vi "Refactor Object for Library Rename.vi"(8 "error in (no error)":errorcluster, 10 "rename data":T2, 11 "object reference in":refnum<vi>) -> (0 "error out":errorcluster, 1 "refactored dependency":bool, 2 "refactor result":T1, 3 "object reference out":refnum<vi>)   [LabVIEW 2021, in "MeasurementService Editor.lvlib"]
uses:
  MeasurementService Editor.lvlib
  Refactor Object Result.ctl
  Rename Refactor Mapping Info.ctl
  Rename Refactor Data.ctl
  Rename String Mapping.ctl
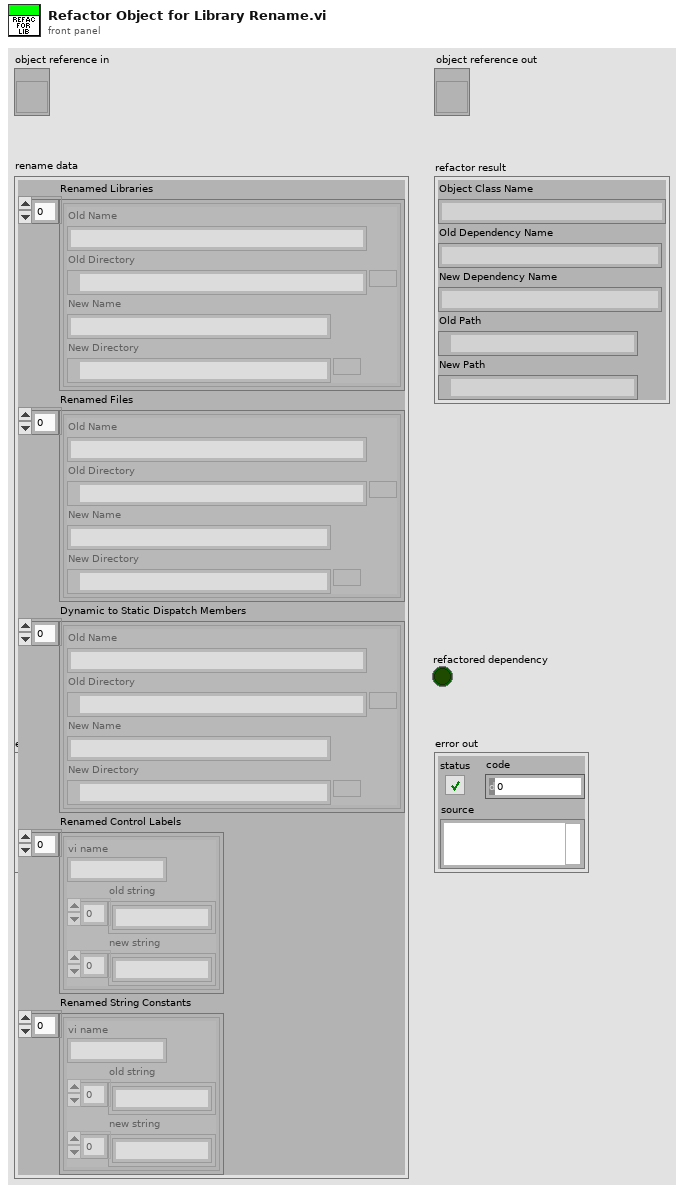
[diagram p1: front panel]
types:
  T1 = typedef "MeasurementService Editor.lvlib/Refactor Object Result.ctl" = cluster{"Object Class Name":string, "Old Dependency Name":string, "New Dependency Name":string, "Old Path":path, "New Path":path}
  T2 = typedef "MeasurementService Editor.lvlib/Rename Refactor Data.ctl" = cluster{"Renamed Libraries":T3[], "Renamed Files":T3[], "Dynamic to Static Dispatch Members":T3[], "Renamed Control Labels":T4[], "Renamed String Constants":T4[]}
  T3 = typedef "MeasurementService Editor.lvlib/Rename Refactor Mapping Info.ctl" = cluster{"Old Name":string, "Old Directory":path, "New Name":string, "New Directory":path}
  T4 = typedef "MeasurementService Editor.lvlib/Rename String Mapping.ctl" = cluster{"vi name":string, "old string":string[], "new string":string[]}
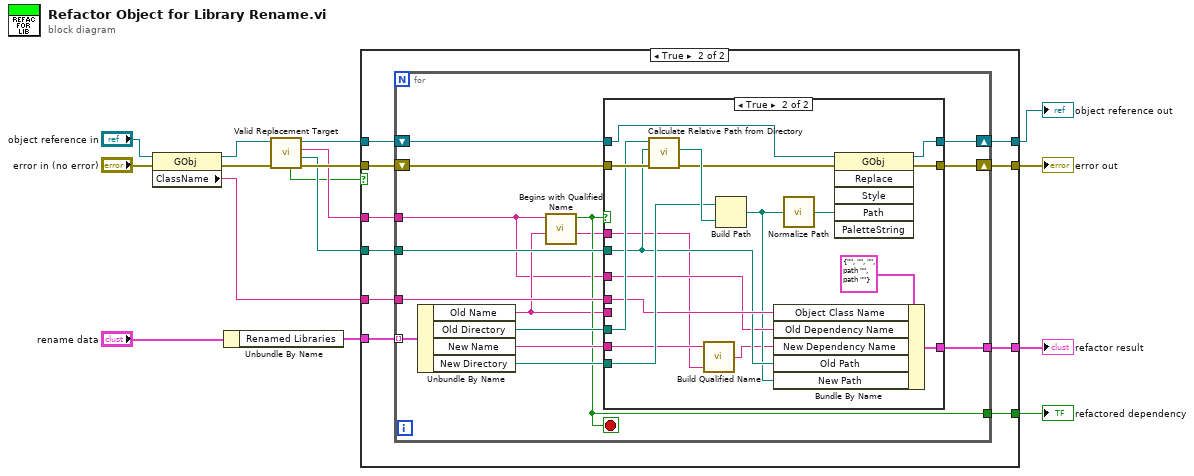
[diagram p0: block diagram]
diagram:
  n1 = property class="GObj"(reference="object reference in", error in="error in (no error)") -> (reference out=w2:refnum<vi>, error out=w7:errorcluster, "ClassName"=w14:string)
  n2 = Unbundle By Name("rename data") -> ("Renamed Libraries"=w13:T3[])
  n3 = call "Valid Replacement Target.vi"("error in (no error)"=w7, "object reference in"=w2) -> ("error out"=w6:errorcluster, "missing path"=w5:path, "missing name"=w4:string, "object reference out"=w1:refnum<vi>, "valid replacement target"=w3:bool)  [unwired: 5 in]
  n4 = case shown="True" w3 {
    tunnel: w1 -> [w17 w28]
    tunnel: w6 -> [w18 w27]
    tunnel: w4 -> [_ w19]
    tunnel: [w18 w22] -> w9
    tunnel: [w17 w23] -> w8
    tunnel: w14 -> [_ w24]
    tunnel: w5 -> [_ w25]
    tunnel: w13 -> [_ w26]
    tunnel: [_ w21] -> w11
    tunnel: [_ w20] -> w10
    frame False {
    }
    frame True {
      n5 = for {
        shift-right: [w39] -> w22
        shift-left: w27 -> [w41]
        shift-right: [w40] -> w23
        shift-left: w28 -> [w42]
        tunnel: w26 -> [w43] mode=indexing
        tunnel: w25 -> [w37]
        tunnel: [w32] -> w21
        tunnel: w24 -> [w35]
        tunnel: [w33] -> w20
        tunnel: w19 -> [w29]
        stop <- w32 stop-if-true
        n6 = Unbundle By Name(w43) -> ("Old Name"=w31:string, "Old Directory"=w38:path, "New Name"=w34:string, "New Directory"=w36:path)
        n7 = call "Begins with Qualified Name.vi"("beginning name"=w31, "name"=w29) -> ("ending name"=w30:string, "begins with name"=w32:bool)  [unwired: 8 in]
        n8 = case shown="True" w32 {
          tunnel: w42 -> [w45 w56]
          tunnel: w41 -> [w44 w63]
          tunnel: [w45 w57] -> w40
          tunnel: [w44 w59] -> w39
          tunnel: w38 -> [_ w62]
          tunnel: w37 -> [_ w53]
          tunnel: w36 -> [_ w60]
          tunnel: w35 -> [_ w54]
          tunnel: w31 -> [_ _]
          tunnel: w34 -> [_ w48]
          tunnel: [_ w52] -> w33
          tunnel: w30 -> [_ w47]
          tunnel: w29 -> [_ w51]
          frame False {
          }
          frame True {
            n9 = call "Calculate Relative Path from Directory.vi"("error in (no error)"=w63, "path"=w53, "directory"=w62) -> ("error out"=w58:errorcluster, "relative path"=w61:path)  [unwired: 7 in]
            n10 = call "Build Qualified Name.vi"("name"=w47, "base name"=w48) -> ("appended name"=w46:string)  [unwired: 3 in]
            n11 = Build Path(base path=w60, name or relative path=w61) -> (appended path=w50:path)
            n12 = Bundle By Name(cluster=T1 {"Object Class Name"="", "Old Dependency Name"="", "New Dependency Name"="", "Old Path"=path "", "New Path"=path ""} ("Rename Refactor Result"), "Object Class Name"=w54, "Old Dependency Name"=w51, "New Dependency Name"=w46, "Old Path"=w53, "New Path"=w50) -> (w52:T1)
            n13 = call "Normalize Path.vi"("path"=w50) -> ("normalized path"=w49:path)
            n14 = invoke class="GObj" method="Replace"(reference=w56, error in=w58, "Path"=w49) -> (reference out=w57:refnum<vi>, error out=w59:errorcluster)  [unwired: 3 in, 4 out]
          }
        }
      }
    }
  }
  "error out" <- w9
  "object reference out" <- w8
  "refactor result" <- w10
  "refactored dependency" <- w11
